vi "MTS_ClearWSTree2.vi"(8 "error in":errorcluster, 11 "Tree Refnum":refnum<vi>) -> (0 "error out":errorcluster, 3 "Tree Refnum (dup)":refnum<vi>)   [LabVIEW 2009]
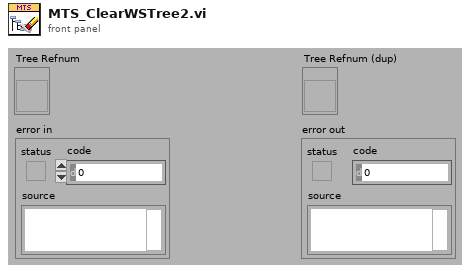
[diagram p1: front panel]
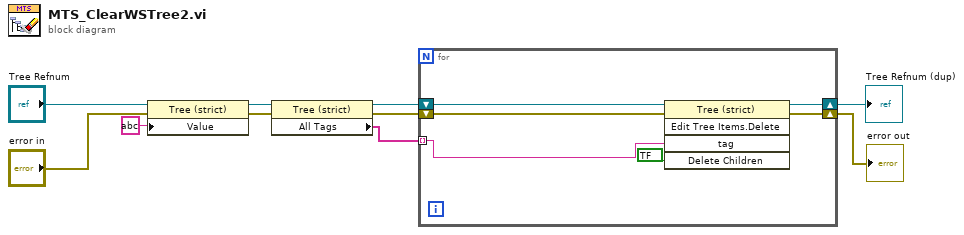
[diagram p0: block diagram]
diagram:
  n1 = property on="Property Node" class="Tree (strict)"(reference="Tree Refnum", error in="error in", "Value"=string ?) -> (reference out=w3:refnum<vi>, error out=w4:errorcluster)
  n2 = property on="Property Node" class="Tree (strict)"(reference=w3, error in=w4) -> (reference out=w8:refnum<vi>, error out=w7:errorcluster, "All Tags"=w6:string[])
  n3 = for {
    tunnel: w6 -> [w14] mode=indexing
    shift-right: [w15] -> w9
    shift-left: w7 -> [w12]
    shift-right: [w16] -> w10
    shift-left: w8 -> [w11]
    n4 = invoke on="Invoke Node" class="Tree (strict)" method="Edit Tree Items.Delete"(reference=w11, error in=w12, "tag"=w14, "Delete Children"=bool ? ("Delete Children?")) -> (reference out=w16:refnum<vi>, error out=w15:errorcluster)  [unwired: 1 in, 3 out]
  }
  "Tree Refnum (dup)" <- w10
  "error out" <- w9
